vi "update hydrolysis feeding.vi"(7 "number_timestamps":i32, 8 "error in (no error)":errorcluster, 9 "amount":string, 10 "time":string, 11 "hydrolysis_specfile":string) -> (0 "error out":errorcluster)   [LabVIEW 2019, in "libFileFunctions.lvlib"]
doc: "void update_hydrolysis_feeding(const char* hydrolysis_specfile, double time[], double amount[], int number_timestamps);"
uses:
  libFileFunctions.lvlib
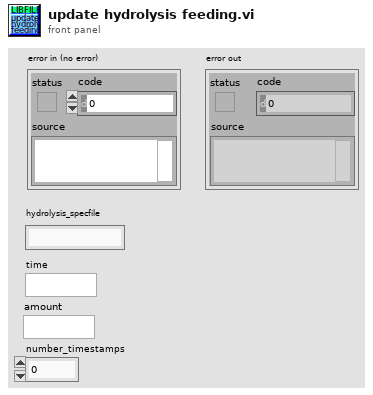
[diagram p1: front panel]
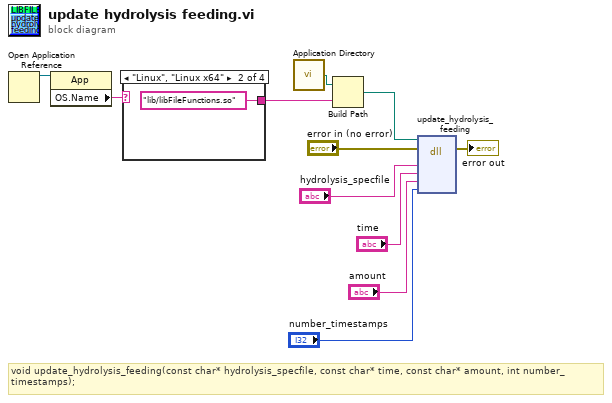
[diagram p0: block diagram]
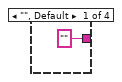
[diagram p2: hidden frame]
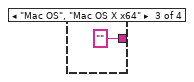
[diagram p3: hidden frame]
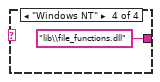
[diagram p4: hidden frame]
diagram:
  # "void update_hydrolysis_feeding(const char* hydrolysis_specfile, const char* time, const char* amount, int number_timestamps);"
  n1 = Open Application Reference() -> (3:w7:refnum<vi>)  [unwired: 4 in, 1 out]
  n2 = property class="App"(reference=w7) -> ("OS.Name"=w6:string)  [unwired: 1 in, 2 out]
  n3 = case shown="\"Linux\", \"Linux x64\"" w6 {
    tunnel: ["" ("return type") "lib/libFileFunctions.so" ("name or relative path") "" ("return type") "lib\\file_functions.dll" ("name or relative path")] -> w5
    frame "", Default {
    }
    frame "Linux", "Linux x64" {
    }
    frame "Mac OS", "Mac OS X x64" {
    }
    frame "Windows NT" {
    }
  }
  n4 = call <vilib>:"Application Directory.vi"() -> ("Application Directory"=w4:path)
  n5 = Build Path(base path=w4, name or relative path=w5) -> (appended path=w3:path)
  n6 = dll-call lib="home/paul/Schreibtisch/Biogas_plant_setup/LabView/lib/libFileFunctions/libFileFunctions.*" fn="update_hydrolysis_feeding"(path in=w3, error in="error in (no error)", "hydrolysis_specfile"="hydrolysis_specfile", "time"="time", "amount"="amount", "number_timestamps"="number_timestamps") -> (error out=→"error out":errorcluster)  [unwired: 6 in, 1 out]
